vi "dfd_Normalized Lattice k.vi"(11 "k":dbl[](array[numeric]) format="%.2f") -> (3 "^k":dbl[](array[numeric]) format="%.2f")   [LabVIEW 2017, in "NI_DigFilterLicensed.lvlib"]
uses:
  <vilib>/addons/Digital Filter Design/NI_DigFilterLicensed.lvlib
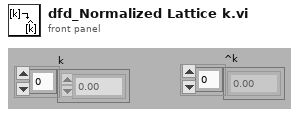
[diagram p1: front panel]
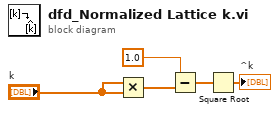
[diagram p0: block diagram]
diagram:
  n1 = Multiply(x="k", y="k") -> (x*y=w1:dbl[])
  n2 = Subtract(x=1.0, y=w1) -> (x-y=w3:dbl[])
  n3 = Square Root(x=w3) -> (sqrt(x)=→"^k":dbl[])
